vi "SL2_AD_DLL_Phoibos_AquireAndGetData.vi"(4 "ignorSync":bool=TRUE, 5 "dwellTime_µs":u32, 6 "error in":errorcluster, 7 "chanId":u32, 8 "pHandle":u32, 9 "dll_path":path) -> (0 "error out":errorcluster, 1 "data":u32[][](array[numeric]), 3 "path out":path)   [LabVIEW 2010]
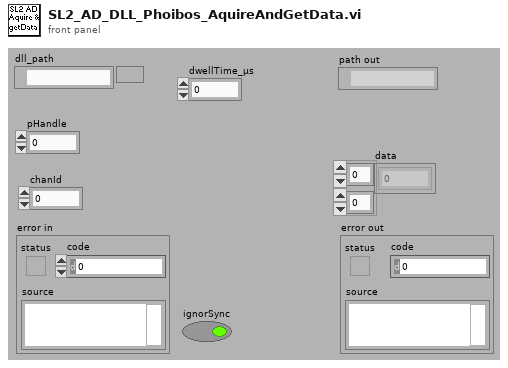
[diagram p1: front panel]
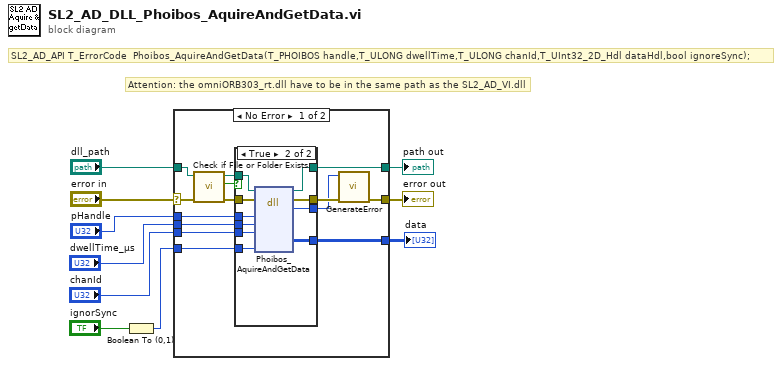
[diagram p0: block diagram]
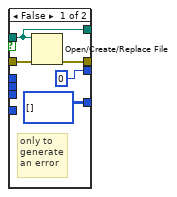
[diagram p2: hidden frame]
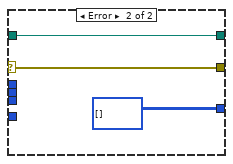
[diagram p3: hidden frame]
diagram:
  # "SL2_AD_API T_ErrorCode  Phoibos_AquireAndGetData(T_PHOIBOS handle,T_ULONG dwellTime,T_ULONG chanId,T_UInt32_2D_Hdl dataHdl,bool ignoreSync);"
  # "Attention: the omniORB303_rt.dll have to be in the same path as the SL2_AD_VI.dll"
  n1 = Boolean To (0,1)(Boolean="ignorSync") -> (0, 1=w2:i16)
  n2 = case shown="No Error" "error in" {
    selector: "error in" -> [w23 w42]
    tunnel: [w15 w42] -> w10
    tunnel: [w24 w41] -> w9
    tunnel: "dll_path" -> [w22 w41]
    tunnel: "pHandle" -> [w21 _]
    tunnel: "dwellTime_µs" -> [w20 _]
    tunnel: "chanId" -> [w19 _]
    tunnel: w2 -> [w18 _]
    tunnel: [w17 u32[][] [] ("data")] -> w1
    frame No Error {
      n3 = call <vilib>:"Check if File or Folder Exists.vi"("error in (no error)"=w23, "path"=w22) -> ("error out"=w13:errorcluster, "file or folder exists?"=w11:bool, "dup path"=w12:path)  [unwired: 7 in]
      n4 = case shown="True" w11 {
        tunnel: [w29 w38] -> w16
        tunnel: [w27 w37] -> w24
        tunnel: w13 -> [w28 w39]
        tunnel: w12 -> [w27 w36]
        tunnel: [u32 0 ("pHandle") w35] -> w14
        tunnel: w21 -> [_ w34]
        tunnel: w20 -> [_ w33]
        tunnel: w19 -> [_ w32]
        tunnel: w18 -> [_ w31]
        tunnel: [u32[][] [] ("data") w30] -> w17
        frame False {
          # "only to generate an error"
          n5 = Open/Create/Replace File(file path (use dialog)=w27, error in=w28) -> (error out=w29:errorcluster)  [unwired: 4 in, 2 out]
        }
        frame True {
          n6 = dll-call lib="C:/Programme/SPECS/SpecsLab2/programming/LabView7.1/SL2_AD_VI.dll" fn="Phoibos_AquireAndGetData" ("AquireData")(path in=w36, error in=w39, "pHandle"=w34, "dwellTime"=w33, "chanId"=w32, "ignoreSync"=w31) -> (path out=w37:path, error out=w38:errorcluster, "errorCode"=w35:u32, "data"=w30:u32[][])  [unwired: 6 in]
        }
      }
      n7 = call "GenerateError.vi"("error in"=w16, "error_code"=w14) -> ("error out"=w15:errorcluster)  [unwired: 9 in]
    }
    frame Error {
    }
  }
  "error out" <- w10
  "path out" <- w9
  "data" <- w1
